vi "MSScript_Exe_Cmd_Calculation.vi"(2 "Ion trap":cluster{"R0":ext, "Z0":ext}, 5 "ValueArray":string[](array[string])) -> (0 "Is a variable?":bool[](array[boolean]), 1 "ErrorBooleanArray":bool[](array[boolean]))   [LabVIEW 2018, in "MSScript.lvclass"]
uses:
  MSScript.lvclass
  Calc/MSScript_Calc_Add.vi
  Calc/MSScript_Calc_Sub.vi
  Calc/MSScript_Calc_Multiply.vi
  Calc/MSScript_Calc_Div.vi
  Calc/MSScript_Calc_Pow.vi
  Calc/MSScript_Calc_Mod.vi
  Calc/MSScript_Calc_Floor.vi
  Calc/MSScript_Calc_Ceil.vi
  Calc/MSScript_Calc_Round.vi
  Calc/MSScript_Calc_Abs.vi
  Calc/MSScript_Calc_Sign.vi
  Calc/MSScript_Calc_Max.vi
  Calc/MSScript_Calc_Min.vi
  Calc/MSScript_Calc_mathieu_mz.vi
  Calc/MSScript_Calc_mathieu_freq.vi
  Calc/MSScript_Calc_mathieu_amp.vi
  Calc/MSScript_Calc_mathieu_beta.vi
  Calc/MSScript_Calc_ArrayInit.vi
  Calc/MSScript_Calc_ArraySeries.vi
  Calc/MSScript_Calc_ArrayLen.vi
  Calc/MSScript_Calc_ArrayAdd.vi
  Calc/MSScript_Calc_ArraySub.vi
  Calc/MSScript_Calc_ArrayMultiply.vi
  Calc/MSScript_Calc_ArrayDiv.vi
  Calc/MSScript_Calc_ArrayPow.vi
  Calc/MSScript_Calc_ArrayRoot.vi
  Calc/MSScript_Calc_ArraySum.vi
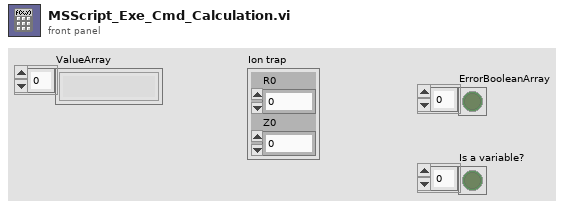
[diagram p1: front panel]
types:
  T1 = enum16{"Scalar", "ScalarArray", "Var", "VarArray", "Error"}
  T2 = typedef "CalcCmdType.ctl" = enum16{"None", "Add", "Sub", "Multiply", "Div", "Pow", "Mod", "Floor", "Ceil", "Round", "Abs", "Sign", "Max", "Min", "mathieu.mz", "mathieu.freq", "mathieu.amp", "mathieu.beta", "ArrayAdd", "ArraySub", "ArrayMultiply", "ArrayDiv", "ArrayPow", "ArrayRoot", "ArrayInit", "ArraySeries", "ArrayLen", "ArraySum"}
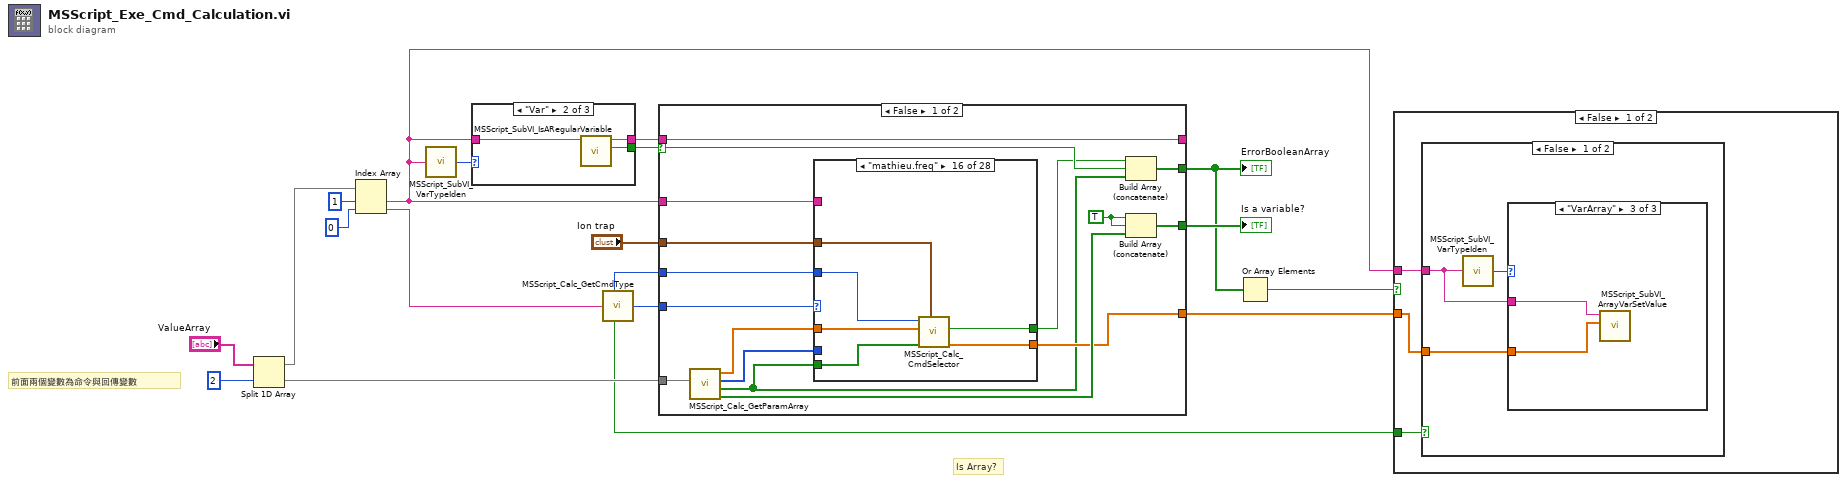
[diagram p0: block diagram]
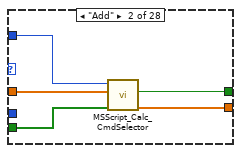
[diagram p3: hidden frame]
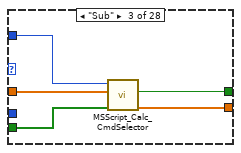
[diagram p4: hidden frame]
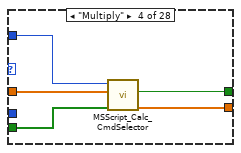
[diagram p5: hidden frame]
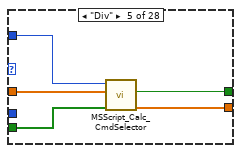
[diagram p6: hidden frame]
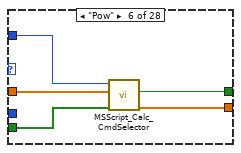
[diagram p7: hidden frame]
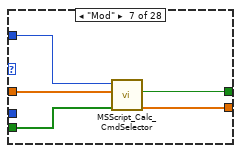
[diagram p8: hidden frame]
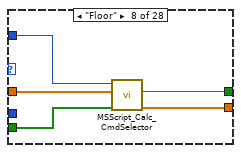
[diagram p9: hidden frame]
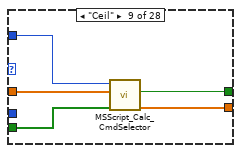
[diagram p10: hidden frame]
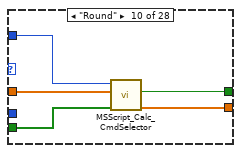
[diagram p11: hidden frame]
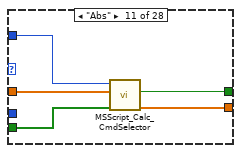
[diagram p12: hidden frame]
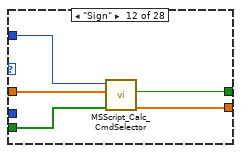
[diagram p13: hidden frame]
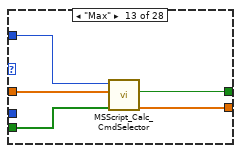
[diagram p14: hidden frame]
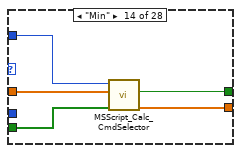
[diagram p15: hidden frame]
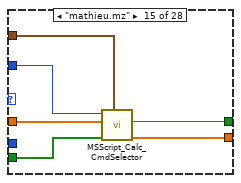
[diagram p16: hidden frame]
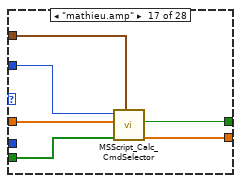
[diagram p17: hidden frame]
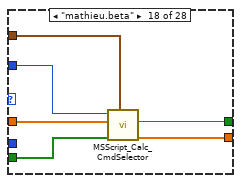
[diagram p18: hidden frame]
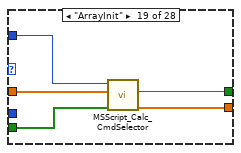
[diagram p19: hidden frame]
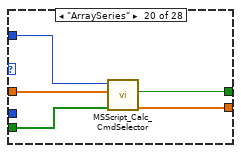
[diagram p20: hidden frame]
diagram:
  # "Is Array?"
  # "前面兩個變數為命令與回傳變數"
  n1 = Split 1D Array(array="ValueArray", index=2 ("y")) -> (first subarray=w17:string[], second subarray=w13:string[])
  n2 = Index Array(array=w17, index #1=1 ("index"), index #2=0 ("index")) -> (element #1=w1:string, element #2=w10:string)
  n3 = call "MSScript_SubVI_VarTypeIden.vi"("Var in"=w1) -> ("Type"=w18:T1)
  n4 = case shown="\"Var\"" w18 {
    tunnel: [w21 w24 w26] -> w11
    tunnel: [TRUE ("irregular") w23 w25] -> w14
    tunnel: w1 -> [w21 w22 w27]
    frame "Scalar", Default {
    }
    frame "Var" {
      n5 = call "MSScript_SubVI_IsARegularVariable.vi"("VarString in"=w22) -> ("irregular"=w23:bool, "VarString out"=w24:string)  [unwired: 6 in, 1 out]
    }
    frame "ScalarArray", "VarArray" {
      n6 = call "MSScript_SubVI_ArraySplit.vi"("VarString in"=w27) -> ("Value Error?"=w25:bool, "@name"=w26:string)  [unwired: 7 in, 2 out]
    }
  }
  n7 = call "MSScript_Calc_GetCmdType.vi"("element"=w10) -> ("Param Items"=w9:i32, "SetArray?"=w3:bool, "Type"=w12:T2)  [unwired: 2 in]
  n8 = case shown="False" w14 {
    selector: w14 -> [w38 w201]
    tunnel: w13 -> [w40 _]
    tunnel: w12 -> [w43 w202]
    tunnel: w11 -> [w30 w195]
    tunnel: w1 -> [w41 _]
    tunnel: [w35 w199] -> w6
    tunnel: [w36 w196] -> w7
    tunnel: w9 -> [w42 _]
    tunnel: [w31 _] -> w4
    tunnel: [w30 w195] -> _
    tunnel: "Ion trap" -> [w28 _]
    frame False {
      w39 = TRUE
      n9 = call "MSScript_Calc_GetParamArray.vi"("Param"=w40) -> ("Is a variable?"=w34:bool[], "Value Error?"=w29:bool[], "Split Index"=w32:i32[], "ArrayVariable out"=w33:ext[])  [unwired: 3 in]
      n10 = case shown="\"mathieu.freq\"" w43 {
        tunnel: w42 -> [_ w48 w53 w58 w63 w68 w73 w78 w83 w88 w93 w98 w103 w108 w114 w120 w126 w132 w137 w142 w147 w154 w161 w168 w175 w182 w189 w194]
        tunnel: w41 -> [_ _ _ _ _ _ _ _ _ _ _ _ _ _ _ _ _ _ _ _ _ w149 w156 w163 w170 w177 w184 _]
        tunnel: [_ w45 w50 w55 w60 w65 w70 w75 w80 w85 w90 w95 w100 w105 w111 w117 w123 w129 w134 w139 w144 w151 w158 w165 w172 w179 w186 w191] -> w37
        tunnel: w33 -> [_ w47 w52 w57 w62 w67 w72 w77 w82 w87 w92 w97 w102 w107 w113 w119 w125 w131 w136 w141 w146 w153 w160 w167 w174 w181 w188 w193]
        tunnel: w32 -> [_ _ _ _ _ _ _ _ _ _ _ _ _ _ _ _ _ _ _ _ _ w148 w155 w162 w169 w176 w183 _]
        tunnel: [_ w44 w49 w54 w59 w64 w69 w74 w79 w84 w89 w94 w99 w104 w110 w116 w122 w128 w135 w140 w145 w150 w157 w164 w171 w178 w185 w190] -> w31
        tunnel: w29 -> [_ w46 w51 w56 w61 w66 w71 w76 w81 w86 w91 w96 w101 w106 w112 w118 w124 w130 w133 w138 w143 w152 w159 w166 w173 w180 w187 w192]
        tunnel: w28 -> [_ _ _ _ _ _ _ _ _ _ _ _ _ _ w109 w115 w121 w127 _ _ _ _ _ _ _ _ _ _]
        frame "None", Default {
        }
        frame "Add" {
          n11 = call-poly "MSScript_Calc_CmdSelector.vi"("Value Error?"=w46, "ArrayVariable in"=w47, "Param Items"=w48) -> ("ArrayVariable out"=w44:ext[], "CmdError?"=w45:bool)  [unwired: 5 in]
        }
        frame "Sub" {
          n12 = call-poly "MSScript_Calc_CmdSelector.vi"("Value Error?"=w51, "ArrayVariable in"=w52, "Param Items"=w53) -> ("ArrayVariable out"=w49:ext[], "CmdError?"=w50:bool)  [unwired: 5 in]
        }
        frame "Multiply" {
          n13 = call-poly "MSScript_Calc_CmdSelector.vi"("Value Error?"=w56, "ArrayVariable in"=w57, "Param Items"=w58) -> ("ArrayVariable out"=w54:ext[], "CmdError?"=w55:bool)  [unwired: 5 in]
        }
        frame "Div" {
          n14 = call-poly "MSScript_Calc_CmdSelector.vi"("Value Error?"=w61, "ArrayVariable in"=w62, "Param Items"=w63) -> ("ArrayVariable out"=w59:ext[], "CmdError?"=w60:bool)  [unwired: 5 in]
        }
        frame "Pow" {
          n15 = call-poly "MSScript_Calc_CmdSelector.vi"("Value Error?"=w66, "ArrayVariable in"=w67, "Param Items"=w68) -> ("ArrayVariable out"=w64:ext[], "CmdError?"=w65:bool)  [unwired: 5 in]
        }
        frame "Mod" {
          n16 = call-poly "MSScript_Calc_CmdSelector.vi"("Value Error?"=w71, "ArrayVariable in"=w72, "Param Items"=w73) -> ("ArrayVariable out"=w69:ext[], "CmdError?"=w70:bool)  [unwired: 5 in]
        }
        frame "Floor" {
          n17 = call-poly "MSScript_Calc_CmdSelector.vi"("Value Error?"=w76, "ArrayVariable in"=w77, "Param Items"=w78) -> ("ArrayVariable out"=w74:ext[], "CmdError?"=w75:bool)  [unwired: 5 in]
        }
        frame "Ceil" {
          n18 = call-poly "MSScript_Calc_CmdSelector.vi"("Value Error?"=w81, "ArrayVariable in"=w82, "Param Items"=w83) -> ("ArrayVariable out"=w79:ext[], "CmdError?"=w80:bool)  [unwired: 5 in]
        }
        frame "Round" {
          n19 = call-poly "MSScript_Calc_CmdSelector.vi"("Value Error?"=w86, "ArrayVariable in"=w87, "Param Items"=w88) -> ("ArrayVariable out"=w84:ext[], "CmdError?"=w85:bool)  [unwired: 5 in]
        }
        frame "Abs" {
          n20 = call-poly "MSScript_Calc_CmdSelector.vi"("Value Error?"=w91, "ArrayVariable in"=w92, "Param Items"=w93) -> ("ArrayVariable out"=w89:ext[], "CmdError?"=w90:bool)  [unwired: 5 in]
        }
        frame "Sign" {
          n21 = call-poly "MSScript_Calc_CmdSelector.vi"("Value Error?"=w96, "ArrayVariable in"=w97, "Param Items"=w98) -> ("ArrayVariable out"=w94:ext[], "CmdError?"=w95:bool)  [unwired: 5 in]
        }
        frame "Max" {
          n22 = call-poly "MSScript_Calc_CmdSelector.vi"("Value Error?"=w101, "ArrayVariable in"=w102, "Param Items"=w103) -> ("ArrayVariable out"=w99:ext[], "CmdError?"=w100:bool)  [unwired: 5 in]
        }
        frame "Min" {
          n23 = call-poly "MSScript_Calc_CmdSelector.vi"("Value Error?"=w106, "ArrayVariable in"=w107, "Param Items"=w108) -> ("ArrayVariable out"=w104:ext[], "CmdError?"=w105:bool)  [unwired: 5 in]
        }
        frame "mathieu.mz" {
          n24 = call-poly "MSScript_Calc_CmdSelector.vi"("Ion trap"=w109, "Value Error?"=w112, "ArrayVariable in"=w113, "Param Items"=w114) -> ("ArrayVariable out"=w110:ext[], "CmdError?"=w111:bool)  [unwired: 4 in]
        }
        frame "mathieu.freq" {
          n25 = call-poly "MSScript_Calc_CmdSelector.vi"("Ion trap"=w115, "Value Error?"=w118, "ArrayVariable in"=w119, "Param Items"=w120) -> ("ArrayVariable out"=w116:ext[], "CmdError?"=w117:bool)  [unwired: 4 in]
        }
        frame "mathieu.amp" {
          n26 = call-poly "MSScript_Calc_CmdSelector.vi"("Ion trap"=w121, "Value Error?"=w124, "ArrayVariable in"=w125, "Param Items"=w126) -> ("ArrayVariable out"=w122:ext[], "CmdError?"=w123:bool)  [unwired: 4 in]
        }
        frame "mathieu.beta" {
          n27 = call-poly "MSScript_Calc_CmdSelector.vi"("Ion trap"=w127, "Value Error?"=w130, "ArrayVariable in"=w131, "Param Items"=w132) -> ("ArrayVariable out"=w128:ext[], "CmdError?"=w129:bool)  [unwired: 4 in]
        }
        frame "ArrayInit" {
          n28 = call-poly "MSScript_Calc_CmdSelector.vi"("Value Error?"=w133, "ArrayVariable in"=w136, "Param Items"=w137) -> ("ArrayVariable out"=w135:ext[], "CmdError?"=w134:bool)  [unwired: 5 in]
        }
        frame "ArraySeries" {
          n29 = call-poly "MSScript_Calc_CmdSelector.vi"("Value Error?"=w138, "ArrayVariable in"=w141, "Param Items"=w142) -> ("ArrayVariable out"=w140:ext[], "CmdError?"=w139:bool)  [unwired: 5 in]
        }
        frame "ArrayLen" {
          n30 = call-poly "MSScript_Calc_CmdSelector.vi"("Value Error?"=w143, "ArrayVariable in"=w146, "Param Items"=w147) -> ("ArrayVariable out"=w145:ext[], "CmdError?"=w144:bool)  [unwired: 5 in]
        }
        frame "ArrayAdd" {
          n31 = call-poly "MSScript_Calc_CmdSelector.vi"("VarString in"=w149, "Value Error?"=w152, "Split Index"=w148, "ArrayVariable in"=w153, "Param Items"=w154) -> ("ArrayVariable out"=w150:ext[], "CmdError?"=w151:bool)  [unwired: 3 in]
        }
        frame "ArraySub" {
          n32 = call-poly "MSScript_Calc_CmdSelector.vi"("VarString in"=w156, "Value Error?"=w159, "Split Index"=w155, "ArrayVariable in"=w160, "Param Items"=w161) -> ("ArrayVariable out"=w157:ext[], "CmdError?"=w158:bool)  [unwired: 3 in]
        }
        frame "ArrayMultiply" {
          n33 = call-poly "MSScript_Calc_CmdSelector.vi"("VarString in"=w163, "Value Error?"=w166, "Split Index"=w162, "ArrayVariable in"=w167, "Param Items"=w168) -> ("ArrayVariable out"=w164:ext[], "CmdError?"=w165:bool)  [unwired: 3 in]
        }
        frame "ArrayDiv" {
          n34 = call-poly "MSScript_Calc_CmdSelector.vi"("VarString in"=w170, "Value Error?"=w173, "Split Index"=w169, "ArrayVariable in"=w174, "Param Items"=w175) -> ("ArrayVariable out"=w171:ext[], "CmdError?"=w172:bool)  [unwired: 3 in]
        }
        frame "ArrayPow" {
          n35 = call-poly "MSScript_Calc_CmdSelector.vi"("VarString in"=w177, "Value Error?"=w180, "Split Index"=w176, "ArrayVariable in"=w181, "Param Items"=w182) -> ("ArrayVariable out"=w178:ext[], "CmdError?"=w179:bool)  [unwired: 3 in]
        }
        frame "ArrayRoot" {
          n36 = call-poly "MSScript_Calc_CmdSelector.vi"("VarString in"=w184, "Value Error?"=w187, "Split Index"=w183, "ArrayVariable in"=w188, "Param Items"=w189) -> ("ArrayVariable out"=w185:ext[], "CmdError?"=w186:bool)  [unwired: 3 in]
        }
        frame "ArraySum" {
          n37 = call-poly "MSScript_Calc_CmdSelector.vi"("Value Error?"=w192, "ArrayVariable in"=w193, "Param Items"=w194) -> ("ArrayVariable out"=w190:ext[], "CmdError?"=w191:bool)  [unwired: 5 in]
        }
      }
      n38 = Build Array (concatenate)(w37, w38, w29) -> (w35:bool[])
      n39 = Build Array (concatenate)(w39, w39, w34) -> (w36:bool[])
    }
    frame True {
      w198 = TRUE
      w197 = bool[] [FALSE] ("array")
      n40 = case shown="\"None\"" w202 {
        tunnel: [TRUE _] -> w200
        frame "None" {
        }
        frame "Add", Default {
        }
      }
      n41 = Build Array (concatenate)(w200, w201, w197) -> (w199:bool[])
      n42 = Build Array (concatenate)(w198, w198, w197) -> (w196:bool[])
    }
  }
  "ErrorBooleanArray" <- w6
  "Is a variable?" <- w7
  n43 = Or Array Elements(Boolean array=w6) -> (logical OR=w5:bool)
  n44 = case shown="False" w5 {
    tunnel: w4 -> [w204 _]
    tunnel: w1 -> [w206 _]
    tunnel: w3 -> [w205 _]
    frame False {
      n45 = case shown="False" w205 {
        tunnel: w206 -> [w207 w218]
        tunnel: w204 -> [w208 w217]
        frame False {
          n46 = call "MSScript_SubVI_VarTypeIden.vi"("Var in"=w207) -> ("Type"=w209:T1)
          n47 = case shown="\"VarArray\"" w209 {
            tunnel: w208 -> [_ w213 w215]
            tunnel: w207 -> [_ w210 w216]
            frame Default {
            }
            frame "Var" {
              n48 = Index Array(array=w213, index=0) -> (element=w211:ext)
              n49 = call "MSScript_SubVI_ScalarVariableAccess.vi"("Function (Read)"=enum16{"Init", "Write", "Read"}."Write", "VarValue"=w211, "VarName"=w210) -> ()  [unwired: 4 in, 3 out]
            }
            frame "VarArray" {
              n50 = call "MSScript_SubVI_ArrayVarSetValue.vi"("ArrayValue in"=w215, "VarString in"=w216) -> ()  [unwired: 8 in, 2 out]
            }
          }
        }
        frame True {
          n51 = call "MSScript_SubVI_ArrayVarSetValue.vi"("ArrayValue in"=w217, "VarString in"=w218) -> ()  [unwired: 8 in, 2 out]
        }
      }
    }
    frame True {
    }
  }
